vi "Duplicate SIM Profile.vi"(8 "error in (no error)":errorcluster, 9 "New Name (\"SIM1-copy\")":string="SIM1-copy", 10 "SIM Profile (\"SIM1\")":string="SIM1", 11 "VISA resource name":refnum<visa-resource-name>) -> (0 "error out":errorcluster, 3 "VISA resource name out":refnum<visa-resource-name>)   [LabVIEW 2015, in "Rohde&Schwarz CMXP Base.lvlib"]
doc: "Creates a SIM profile with a new name as a copy of the profile with the specified name.\n\nAttribute:\n-\n\nRemote-control command:\nCOPY:SIMProfile"
uses:
  <instrlib>/Rohde&Schwarz CMXP Base/Rohde&Schwarz CMXP Base.lvlib
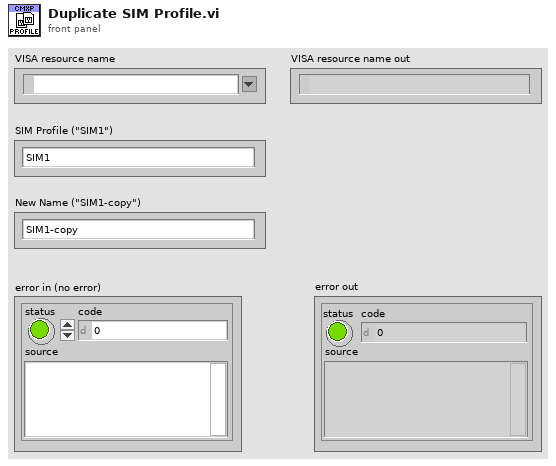
[diagram p1: front panel]
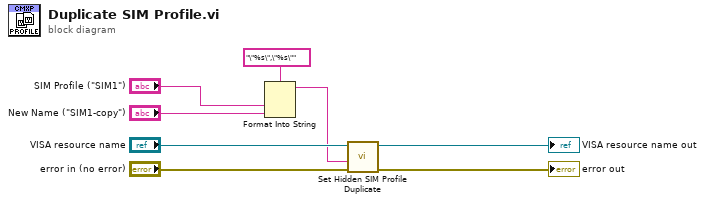
[diagram p0: block diagram]
diagram:
  n1 = Format Into String(format string="\"%s\",\"%s\"", "SIM Profile (\"SIM1\")", "New Name (\"SIM1-copy\")") -> (resulting string=w1:string)  [unwired: 2 in, 1 out]
  n2 = call "Set Hidden SIM Profile Duplicate"("error in (no error)"="error in (no error)", "Hidden SIM Profile Duplicate ()"=w1, "instrument handle"="VISA resource name") -> ("error out"=→"error out":errorcluster, "instrument handle out"=→"VISA resource name out":refnum<visa-resource-name>)  [unwired: 7 in]
